vi "Lookup SharedString.vi"(8 "error in":errorcluster, 10 "Index":string, 11 "SpreadsheetDoc in":refnum<k24>) -> (0 "error out":errorcluster, 2 "String Value":string, 3 "SpreadsheetDoc out":refnum<k24>)   [LabVIEW 2019, in "Open Xml.lvlib"]
uses:
  Open Xml.lvlib
  D:/git/Open-Xml-LabVIEW/Source/DocumentFormat.OpenXml.Framework.dll
  DocumentFormat.OpenXml.Framework.dll
  D:/git/Open-Xml-LabVIEW/Source/DocumentFormat.OpenXml.dll
  DocumentFormat.OpenXml.dll
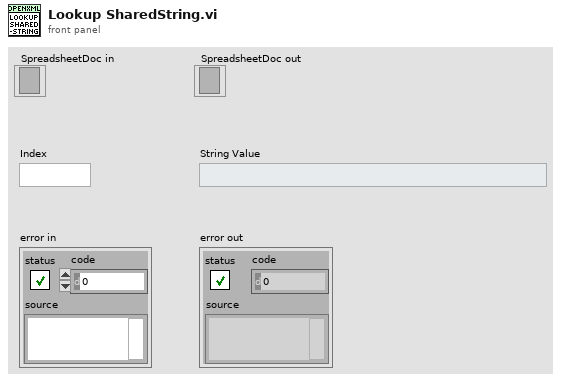
[diagram p1: front panel]
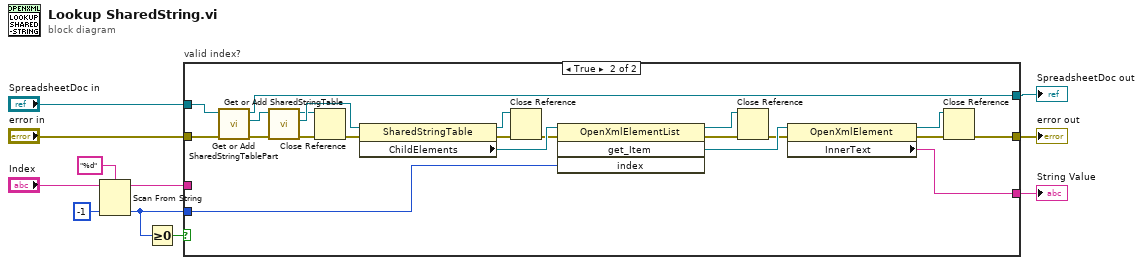
[diagram p0: block diagram]
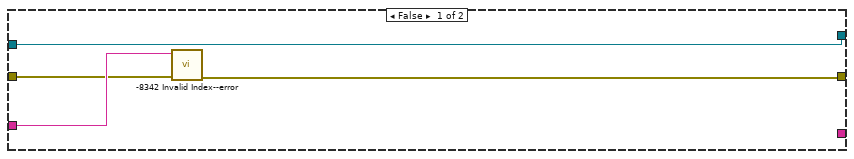
[diagram p2: hidden frame]
diagram:
  n1 = Scan From String(format string="%d", input string="Index", default 1=-1) -> (remaining string=w5:string, output 1=w7:i32)  [unwired: 2 in, 2 out]
  n2 = Greater Or Equal To 0?(x=w7) -> (x >= 0?=w8:bool)
  n3 = case "valid index?" shown="True" w8 {
    tunnel: w7 -> [_ w36]
    tunnel: [w15 w32] -> w6
    tunnel: w5 -> [w14 _]
    tunnel: "SpreadsheetDoc in" -> [w12 w24]
    tunnel: "error in" -> [w13 w23]
    tunnel: [_ w34] -> w2
    tunnel: [w12 w18] -> w1
    frame False {
      n4 = call "-8342 Invalid Index--error.vi"("error in"=w13, "Index"=w14) -> ("error out"=w15:errorcluster)  [unwired: 9 in]
    }
    frame True {
      n5 = call "Get or Add SharedStringTablePart.vi"("error in"=w23, "SpreadsheetDoc in"=w24) -> ("error out"=w22:errorcluster, "SharedStringTablePart"=w21:refnum<k24>, "SpreadsheetDoc out"=w18:refnum<k24>)  [unwired: 7 in]
      n6 = call "Get or Add SharedStringTable.vi"("error in"=w22, "SharedStringTablePart in"=w21) -> ("error out"=w19:errorcluster, "SharedStringTable"=w20:refnum<k24>, "SharedStringTablePart out"=w16:refnum<k24>)  [unwired: 7 in]
      n7 = Close Reference(reference=w16, error in (no error)=w19) -> (error out=w17:errorcluster)
      n8 = property class="SharedStringTable"(reference=w20, error in=w17) -> (reference out=w27:refnum<k24>, error out=w29:errorcluster, "ChildElements"=w37:refnum<k24>)
      n9 = Close Reference(reference=w27, error in (no error)=w29) -> (error out=w28:errorcluster)
      n10 = invoke class="OpenXmlElementList" method="get_Item"(reference=w37, error in=w28, "index"=w36) -> (reference out=w25:refnum<k24>, error out=w35:errorcluster, "get_Item"=w31:refnum<k24>)  [unwired: 1 in, 1 out]
      n11 = Close Reference(reference=w25, error in (no error)=w35) -> (error out=w26:errorcluster)
      n12 = property class="OpenXmlElement"(reference=w31, error in=w26) -> (reference out=w30:refnum<k24>, error out=w33:errorcluster, "InnerText"=w34:string)
      n13 = Close Reference(reference=w30, error in (no error)=w33) -> (error out=w32:errorcluster)
    }
  }
  "error out" <- w6
  "String Value" <- w2
  "SpreadsheetDoc out" <- w1
